vi "GenerateCmdEvent.vi"(8 "error in (no error)":errorcluster, 9 "DATA":variant, 10 "CMD":string, 11 "GUI in":refnum<class "GUI.lvclass">) -> (0 "error out":errorcluster, 3 "GUI out":refnum<class "GUI.lvclass">)   [LabVIEW 2019, in "GUI.lvclass"]
uses:
  GUI.lvclass
  CmdData.ctl
  GUI.lvclass/GUI.ctl
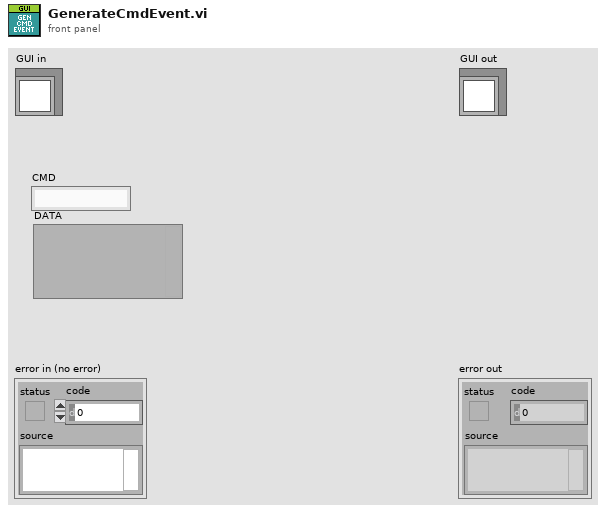
[diagram p1: front panel]
types:
  T1 = typedef "GUI.lvclass/CmdData.ctl" = cluster{"CMD":string, "DATA":variant}
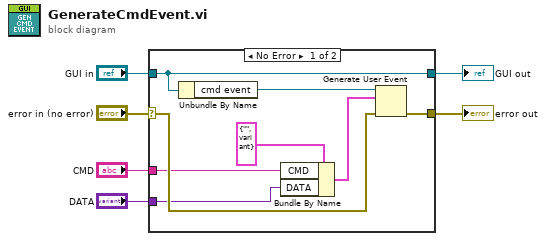
[diagram p0: block diagram]
diagram:
  n1 = case shown="No Error" "error in (no error)" {
    selector: "error in (no error)" -> [w10 w16]
    tunnel: [w9 w16] -> w5
    tunnel: [w13 w15] -> w3
    tunnel: "GUI in" -> [w13 w15]
    tunnel: "CMD" -> [w8 _]
    tunnel: "DATA" -> [w7 _]
    frame No Error {
      n2 = Unbundle By Name(w13) -> ("cmd event"=w14:refnum<user-event>)
      n3 = Bundle By Name(cluster=T1 {"CMD"="", "DATA"=variant} ("event data"), "CMD"=w8, "DATA"=w7) -> (w11:T1)
      n4 = Generate User Event(user event=w14, event data cluster=w11, error in=w10) -> (error out=w9:errorcluster)  [unwired: 1 in, 1 out]
    }
    frame Error {
    }
  }
  "error out" <- w5
  "GUI out" <- w3
